vi "Stop Server.vi"(8 "error in (no error)":errorcluster, 11 "gRPC Server in":refnum<class "Simple_server.lvclass">) -> (0 "error out":errorcluster)   [LabVIEW 2019, in "Simple_server.lvlib" / "Simple_server.lvclass"]
uses:
  Simple_server.lvclass
  Simple_server.lvclass/Simple_server.ctl
  <vilib>/gRPC/LabVIEW gRPC Library/gprc-lvsupport-release.lvlib
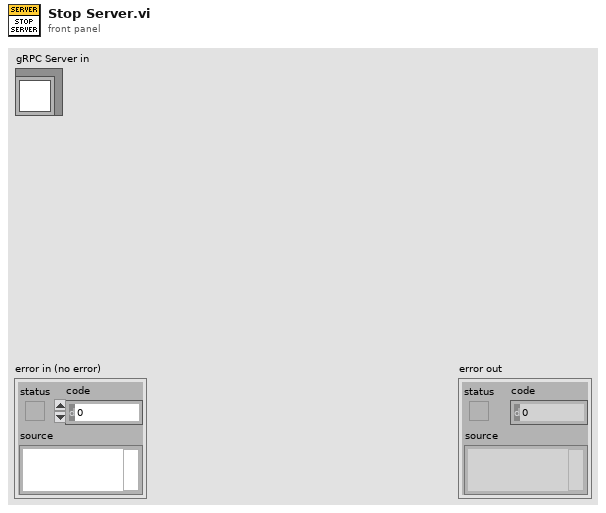
[diagram p1: front panel]
types:
  T1 = typedef "gprc-lvsupport-release.lvlib/grpcId.ctl" = u64
  T2 = typedef "Simple_server.lvlib/Simple_server.lvclass/Server gRPC UEs.ctl" = cluster{"hello_hi gRPC UE":refnum<user-event>}
  T3 = typedef "Simple_server.lvlib/Simple_server.lvclass/Server Internal UEs.ctl" = cluster{"hello_hi Internal UE":refnum<user-event>}
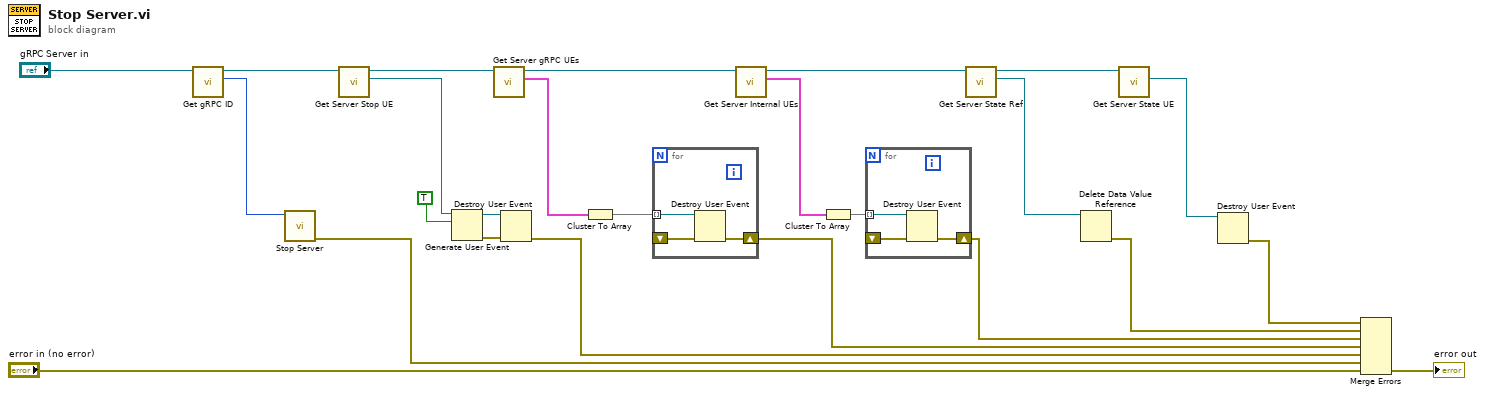
[diagram p0: block diagram]
diagram:
  n1 = call "Get gRPC ID.vi"("OOP Server in"="gRPC Server in") -> ("gRPC ID"=w24:T1, "OOP Server out"=w23:refnum<class "Simple_server.lvclass">)  [unwired: 9 in]
  n2 = call <vilib>:"Stop Server.vi"("Server Id"=w24) -> ("error out"=w11:errorcluster)  [unwired: 10 in]
  n3 = call "Get Server Stop UE.vi"("OOP Server in"=w23) -> ("Server Stop"=w7:refnum<user-event>, "OOP Server out"=w22:refnum<class "Simple_server.lvclass">)  [unwired: 9 in]
  n4 = Generate User Event(user event=w7, event data cluster=TRUE ("event data")) -> (user event out=w8:refnum<user-event>, error out=w9:errorcluster)  [unwired: 2 in]
  n5 = call "Get Server gRPC UEs.vi"("OOP Server in"=w22) -> ("Server RPC Methods"=w20:T2, "OOP Server out"=w21:refnum<class "Simple_server.lvclass">)  [unwired: 9 in]
  n6 = Destroy User Event(user event=w8, error in=w9) -> (error out=w12:errorcluster)
  n7 = Cluster To Array(cluster=w20) -> (array=w19:refnum<user-event>[])
  n8 = for {
    tunnel: w19 -> [w28] mode=indexing
    shift-right: [w26] -> w13
    shift-left: _ -> [w27]
    n9 = Destroy User Event(user event=w28, error in=w27) -> (error out=w26:errorcluster)
  }
  n10 = call "Get Server Internal UEs.vi"("OOP Server in"=w21) -> ("Server Internal UEs"=w18:T3, "OOP Server out"=w6:refnum<class "Simple_server.lvclass">)  [unwired: 9 in]
  n11 = Cluster To Array(cluster=w18) -> (array=w17:refnum<user-event>[])
  n12 = for {
    tunnel: w17 -> [w31] mode=indexing
    shift-right: [w29] -> w14
    shift-left: _ -> [w30]
    n13 = Destroy User Event(user event=w31, error in=w30) -> (error out=w29:errorcluster)
  }
  n14 = call "Get Server State Ref.vi"("Template Server in"=w6) -> ("Server State Ref"=w4:refnum<data-value>, "Template Server out"=w5:refnum<class "Simple_server.lvclass">)  [unwired: 9 in]
  n15 = Delete Data Value Reference(data value reference=w4) -> (error out=w2:errorcluster)  [unwired: 1 in, 1 out]
  n16 = call "Get Server State UE.vi"("Template Server in"=w5) -> ("Server Internal State UE"=w3:refnum<user-event>)  [unwired: 9 in, 1 out]
  n17 = Destroy User Event(user event=w3) -> (error out=w1:errorcluster)  [unwired: 1 in]
  n18 = Merge Errors(w1, w2, w14, w13, w12, w11, "error in (no error)") -> (→"error out":errorcluster)
